vi "Perform Action.vi"(8 "Error In":errorcluster, 10 "Input":variant, 11 "reference in":refnum<class "Voltmeter Virtual CFG.lvclass">) -> (0 "Error Out":errorcluster, 2 "Output":variant, 3 "reference out":refnum<class "Voltmeter Virtual CFG.lvclass">)   [LabVIEW 2023, in "Voltmeter Virtual.lvlib" / "Voltmeter Virtual CFG.lvclass"]
uses:
  Voltmeter Virtual CFG.lvclass
  Voltmeter Virtual CFG.lvclass/Voltmeter Virtual CFG.ctl
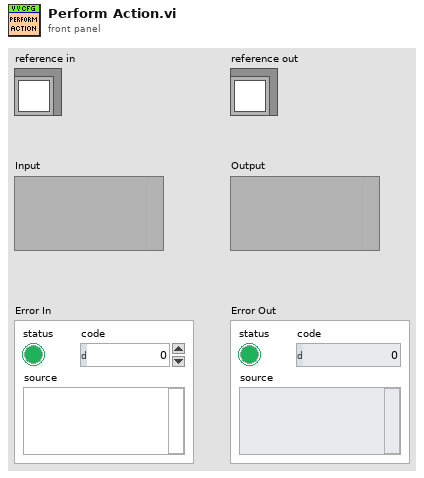
[diagram p1: front panel]
types:
  T1 = typedef "Voltmeter Virtual.lvlib/Voltmeter Virtual CFG.lvclass/ObjectAttributes.ctl" = cluster{"Attribute1":dbl}
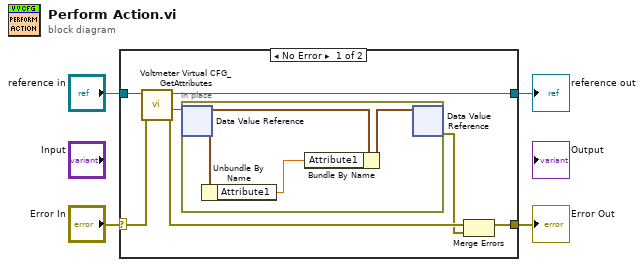
[diagram p0: block diagram]
diagram:
  n1 = case shown="No Error" "Error In" {
    selector: "Error In" -> [w10 w16]
    tunnel: [w9 w16] -> w3
    tunnel: [w8 w15] -> w1
    tunnel: "reference in" -> [w11 w15]
    frame No Error {
      n2 = call "Voltmeter Virtual CFG_GetAttributes.vi"("Error In"=w10, "reference in"=w11) -> ("Error Out"=w6:errorcluster, "DataRef"=w7:refnum<data-value>, "reference out"=w8:refnum<class "Voltmeter Virtual CFG.lvclass">)  [unwired: 6 in, 1 out]
      n3 = in-place {
        n4 = in-place-dvr #1(w7) -> (w13:T1)  [unwired: 1 out]
        n5 = Unbundle By Name(w13) -> ("Attribute1"=w12:dbl)
        n6 = Bundle By Name(cluster=w13, "Attribute1"=w12) -> (w14:T1)
        n7 = in-place-dvr #1(w14) -> (w5:errorcluster)  [unwired: 1 out]
      }
      n8 = Merge Errors(w6, w5) -> (w9:errorcluster)
    }
    frame Error {
    }
  }
  "Error Out" <- w3
  "reference out" <- w1
